vi "New SenseHat.Display.vi"(8 "error in (no error)":errorcluster, 11 "SenseHat in":refnum<class "SenseHat.lvclass">) -> (0 "error out":errorcluster, 3 "SenseHat out":refnum<class "SenseHat.lvclass">)   [LabVIEW 2020, in "RPI.SenseHat.lvlib" / "SenseHat.lvclass"]
doc: "Create and initialize a new RPI.SenseHat.Display object."
uses:
  SenseHat.lvclass
  SenseHat.lvclass/SenseHat.ctl
  RPI.SenseHat.Display/Classes/SenseHat.Display/RPI.SenseHat.Display.lvclass
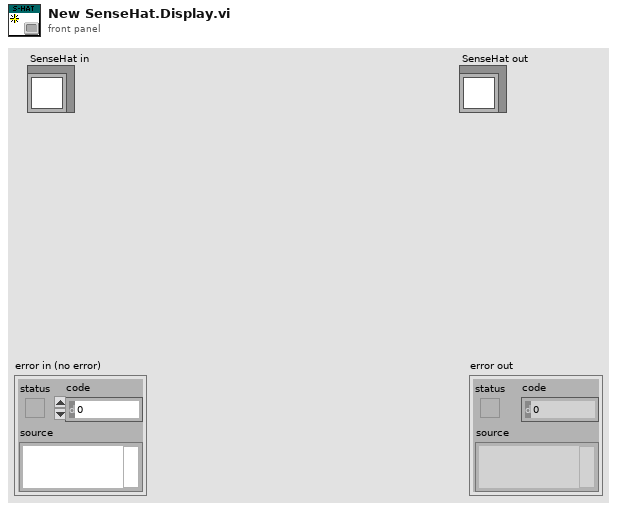
[diagram p1: front panel]
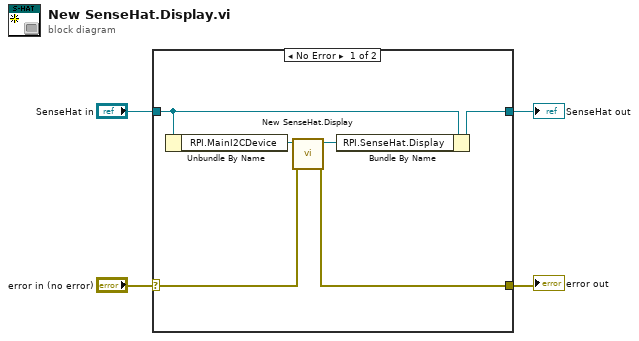
[diagram p0: block diagram]
diagram:
  n1 = case shown="No Error" "error in (no error)" {
    selector: "error in (no error)" -> [w6 w12]
    tunnel: [w5 w12] -> w3
    tunnel: [w9 w11] -> w1
    tunnel: "SenseHat in" -> [w10 w11]
    frame No Error {
      n2 = Unbundle By Name(w10) -> ("RPI.MainI2CDevice"=w8:refnum<class "mainI2CDevice.lvclass">)
      n3 = call "New SenseHat.Display.vi"("error in (no error)"=w6, "MainI2CDevice"=w8) -> ("error out"=w5:errorcluster, "senseHatDisplay out"=w7:refnum<class "RPI.SenseHat.Display.lvclass">)  [unwired: 8 in]
      n4 = Bundle By Name(cluster=w10, "RPI.SenseHat.Display"=w7) -> (w9:refnum<class "SenseHat.lvclass">)
    }
    frame Error {
    }
  }
  "error out" <- w3
  "SenseHat out" <- w1
